vi "Role Status.vi"(8 "error in (no error)":errorcluster, 11 "GUI Manager Module in":refnum<class "GUI Manager Module.lvclass">) -> (0 "error out":errorcluster, 1 "Roles Active":bool, 2 "Role Status":T1, 3 "GUI Manager Module out":refnum<class "GUI Manager Module.lvclass">)   [LabVIEW 2020, in "VolatusGUI.lvlib" / "GUI Manager Module.lvclass"]
uses:
  GUI Manager Module.lvclass
  GUI Manager Module.lvclass/GUI Manager Module.ctl
  Volatus/Roles API/Roles API.lvclass
panel:
  # "Role"
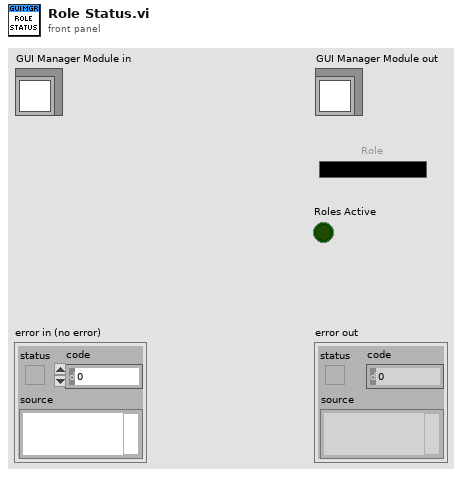
[diagram p1: front panel]
types:
  T1 = cluster{"Color":u32, "Role":string, "Select Role":bool}
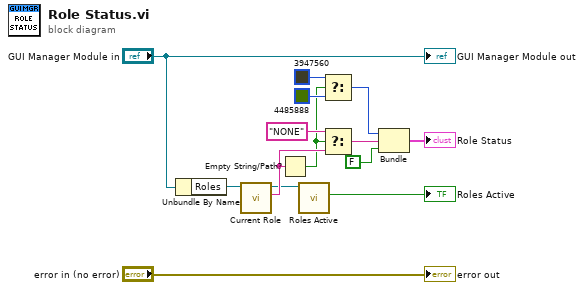
[diagram p0: block diagram]
diagram:
  n1 = Unbundle By Name("GUI Manager Module in") -> ("Roles"=w12:refnum<class "Roles API.lvclass">)
  n2 = call "Current Role.vi"("Roles API in"=w12) -> ("Current Role"=w11:string, "Roles API out"=w2:refnum<class "Roles API.lvclass">)  [unwired: 8 in, 1 out]
  n3 = Empty String/Path?(string/path=w11) -> (empty?=w7:bool)
  n4 = call "Roles Active.vi"("Roles API in"=w2) -> ("Roles Active"=→"Roles Active":bool)  [unwired: 8 in, 2 out]
  n5 = Select(t=u32 3947560, s=w7, f=u32 4485888) -> (s? t:f=w6:u32)
  n6 = Select(t="NONE", s=w7, f=w11) -> (s? t:f=w5:string)
  n7 = Bundle(w6, "Current Role"=w5, FALSE) -> (→"Role Status":cluster{u32, "Current Role":string, bool})  [unwired: 1 in]
  "error out" <- "error in (no error)"
  "GUI Manager Module out" <- "GUI Manager Module in"
